vi "match info fg.vi"(0 "Menu (Set)":enum16{"Get", "Set"}(ring)=enum."Set", 1 "Match Info":T1={"Autonomous Elapsed Seconds"=0.0, "TeleOp Elapsed Seconds"=0.0, "Disabled Elapsed Seconds"=0.0, "Visited Autonomous"=FALSE, "Visited TeleOp"=FALSE, "Visited Disabled"=FALSE, "Autonomous Settings"={"Autonomous Style"=enum."Independent", "VI Refnum"=refnum}}) -> (8 "TeleOp Elapsed Seconds":dbl)   [LabVIEW 2013]
uses:
  <vilib>/Rock Robotics/WPI/DriverStation/WPI_DriverStationMatch Info.ctl
panel:
  # "Get Match Info and Store It"
  # "see, you can just set it easily"
  # "very inconspicuously"
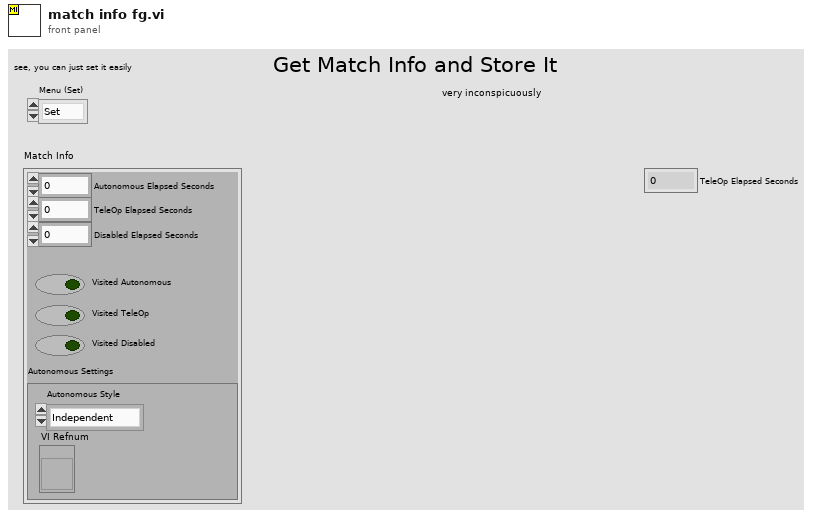
[diagram p1: front panel]
types:
  T1 = typedef "WPI_DriverStationMatch Info.ctl" = cluster{"Autonomous Elapsed Seconds":dbl, "TeleOp Elapsed Seconds":dbl, "Disabled Elapsed Seconds":dbl, "Visited Autonomous":bool, "Visited TeleOp":bool, "Visited Disabled":bool, "Autonomous Settings":cluster{"Autonomous Style":enum16{"Iterative", "Independent"}, "VI Refnum":refnum<vi>}}
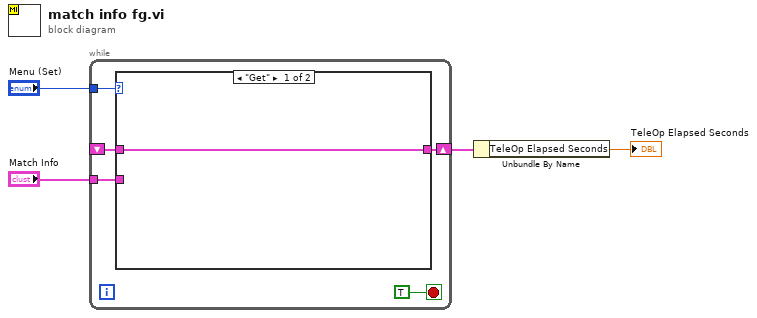
[diagram p0: block diagram]
diagram:
  n1 = while {
    tunnel: "Menu (Set)" -> [w8]
    tunnel: "Match Info" -> [w7]
    shift-right: [w6] -> w2
    shift-left: _ -> [w5]
    stop <- TRUE stop-if-true
    n2 = case shown="\"Get\"" w8 {
      tunnel: w7 -> [_ w11]
      tunnel: [w10 w11] -> w6
      tunnel: w5 -> [w10 _]
      frame "Get" {
      }
      frame "Set", Default {
      }
    }
  }
  n3 = Unbundle By Name(w2) -> ("TeleOp Elapsed Seconds"=→"TeleOp Elapsed Seconds":dbl)
